vi "BeginDrive.vi"() -> (0 "Error Out List":errorcluster[](array[cluster]))   [LabVIEW 2012]
uses:
  <vilib>/Rock Robotics/SystemInterfaces/DIO/FPGA_DIOPWMChannel.ctl
  <vilib>/Rock Robotics/SystemInterfaces/DIO/FPGA_DIOChannel.ctl
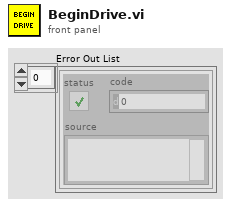
[diagram p1: front panel]
types:
  T1 = typedef "FPGA_DIOChannel.ctl" = enum8{"DIO 1", "DIO 2", "DIO 3", "DIO 4", "DIO 5", "DIO 6", "DIO 7", "DIO 8", "DIO 9", "DIO 10", "DIO 11", "DIO 12", "DIO 13", "DIO 14", "Invalid"}
  T2 = typedef "FPGA_DIOPWMChannel.ctl" = enum8{"PWM 1", "PWM 2", "PWM 3", "PWM 4", "PWM 5", "PWM 6", "PWM 7", "PWM 8", "PWM 9", "PWM 10", "Invalid"}
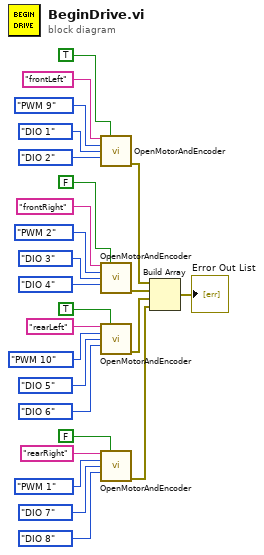
[diagram p0: block diagram]
diagram:
  n1 = call "OpenMotorAndEncoder.vi"("Name"="frontLeft", "Invert"=TRUE, "Motor Channel"=FPGA_DIOPWMChannel."PWM 9", "Encoder A Channel"=FPGA_DIOChannel."DIO 1", "Encoder B Channel"=FPGA_DIOChannel."DIO 2") -> ("error out"=w9:errorcluster)  [unwired: 10 in]
  n2 = call "OpenMotorAndEncoder.vi"("Name"="frontRight", "Invert"=FALSE, "Motor Channel"=FPGA_DIOPWMChannel."PWM 2", "Encoder A Channel"=FPGA_DIOChannel."DIO 3", "Encoder B Channel"=FPGA_DIOChannel."DIO 4") -> ("error out"=w8:errorcluster)  [unwired: 10 in]
  n3 = call "OpenMotorAndEncoder.vi"("Name"="rearLeft", "Invert"=TRUE, "Motor Channel"=FPGA_DIOPWMChannel."PWM 10", "Encoder A Channel"=FPGA_DIOChannel."DIO 5", "Encoder B Channel"=FPGA_DIOChannel."DIO 6") -> ("error out"=w7:errorcluster)  [unwired: 10 in]
  n4 = call "OpenMotorAndEncoder.vi"("Name"="rearRight", "Invert"=FALSE, "Motor Channel"=FPGA_DIOPWMChannel."PWM 1", "Encoder A Channel"=FPGA_DIOChannel."DIO 7", "Encoder B Channel"=FPGA_DIOChannel."DIO 8") -> ("error out"=w6:errorcluster)  [unwired: 10 in]
  n5 = Build Array(w9, w8, w7, w6) -> (→"Error Out List":errorcluster[])
